vi "FG - dCVT DVR - DAQDict.vi"(2 "dCVT DAQDict":T1, 3 "error in (no error)":errorcluster, 4 "Action (Get)":enum16{"Init", "Get", "Set"}(ring)=enum."Get") -> (9 "dCVT DAQDict out":T1, 10 "error out":errorcluster)   [LabVIEW 2020, in "DAQDict.lvlib"]
doc: "Developed by Kevin Thompson\nkevin@thompsonengineering.net\n\nCopyright 2021\nThompson Engineering, LLC"
uses:
  DAQDict.lvlib
  <vilib>/TELLC/Dynamic CVT API/TD Dynamic CVT DVR--ref.ctl
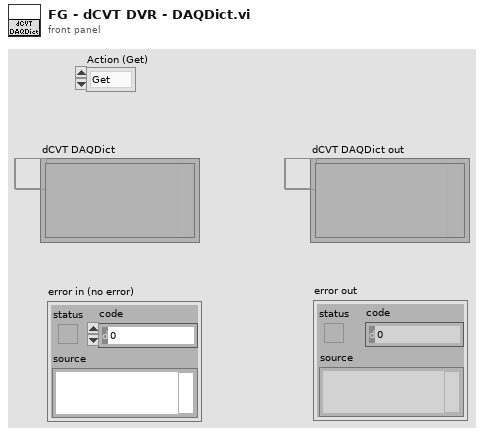
[diagram p1: front panel]
types:
  T1 = typedef "TD Dynamic CVT DVR--ref.ctl" = refnum<data-value>
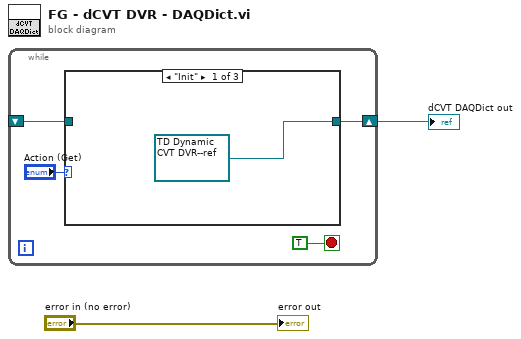
[diagram p0: block diagram]
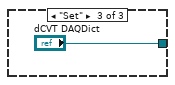
[diagram p3: hidden frame]
diagram:
  n1 = while {
    shift-right: [w4] -> w1
    shift-left: _ -> [w3]
    stop <- TRUE stop-if-true
    n2 = case shown="\"Init\"" "Action (Get)" {
      tunnel: [T1 refnum ("dCVT DVR") w8 "dCVT DAQDict"] -> w4
      tunnel: w3 -> [_ w8 _]
      frame "Init" {
      }
      frame "Get", Default {
      }
      frame "Set" {
      }
    }
  }
  "dCVT DAQDict out" <- w1
  "error out" <- "error in (no error)"
